vi "Go.vi"(9 "Timing Data":T1(array[cluster]), 10 "Control In":T2={"I-O.lvclass"=refnum, "Gantry"=refnum, "Dispenser"="COM1"}, 11 "C4 Dispense in":refnum<class "Iterative Dispense.lvclass">) -> (2 "Control Out":T2={"I-O.lvclass"=refnum, "Gantry"=refnum, "Dispenser"="COM1"}, 3 "C4 Dispense Out":refnum<class "Iterative Dispense.lvclass">)   [LabVIEW 2020, in "Iterative Dispense.lvclass"]
uses:
  Iterative Dispense.lvclass
  Controller/Controllers.ctl
  Controller/I-O/I-O.lvclass
  C:/Program Files (x86)/Aerotech/A3200/LabVIEW/2010/Bin/Aerotech.A3200.dll
  Program Files (x86)/Aerotech/A3200/LabVIEW/2010/Bin/Aerotech.A3200.dll
  Iterative Dispense.lvclass/Iterative Dispense.ctl
  Controller/Motion/A3200/A3200.lvclass
  Controller/Dispenser/Dispenser.lvclass
  Controller/Motion/Motion.lvclass
  Controller/Controller.lvclass
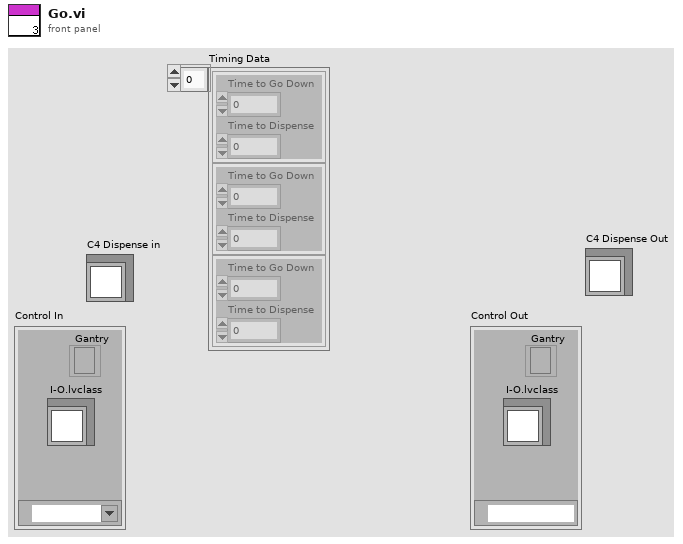
[diagram p1: front panel]
types:
  T1 = cluster{"Time to Go Down":i32, "Time to Dispense":i32}[]
  T2 = typedef "Controller.lvclass/Controllers.ctl" = cluster{"I-O.lvclass":refnum<class "I-O.lvclass">, "Gantry":refnum<k24>, "Dispenser":refnum<visa-resource-name>}
  T3 = typedef "Iterative Dispense.lvclass/Glue Step Enum.ctl" = enum16{"Baseplate to Kapton", "Kapton to Sensor"}
  T4 = cluster{"Time to Go Down":dbl, "Time to Dispense":dbl}
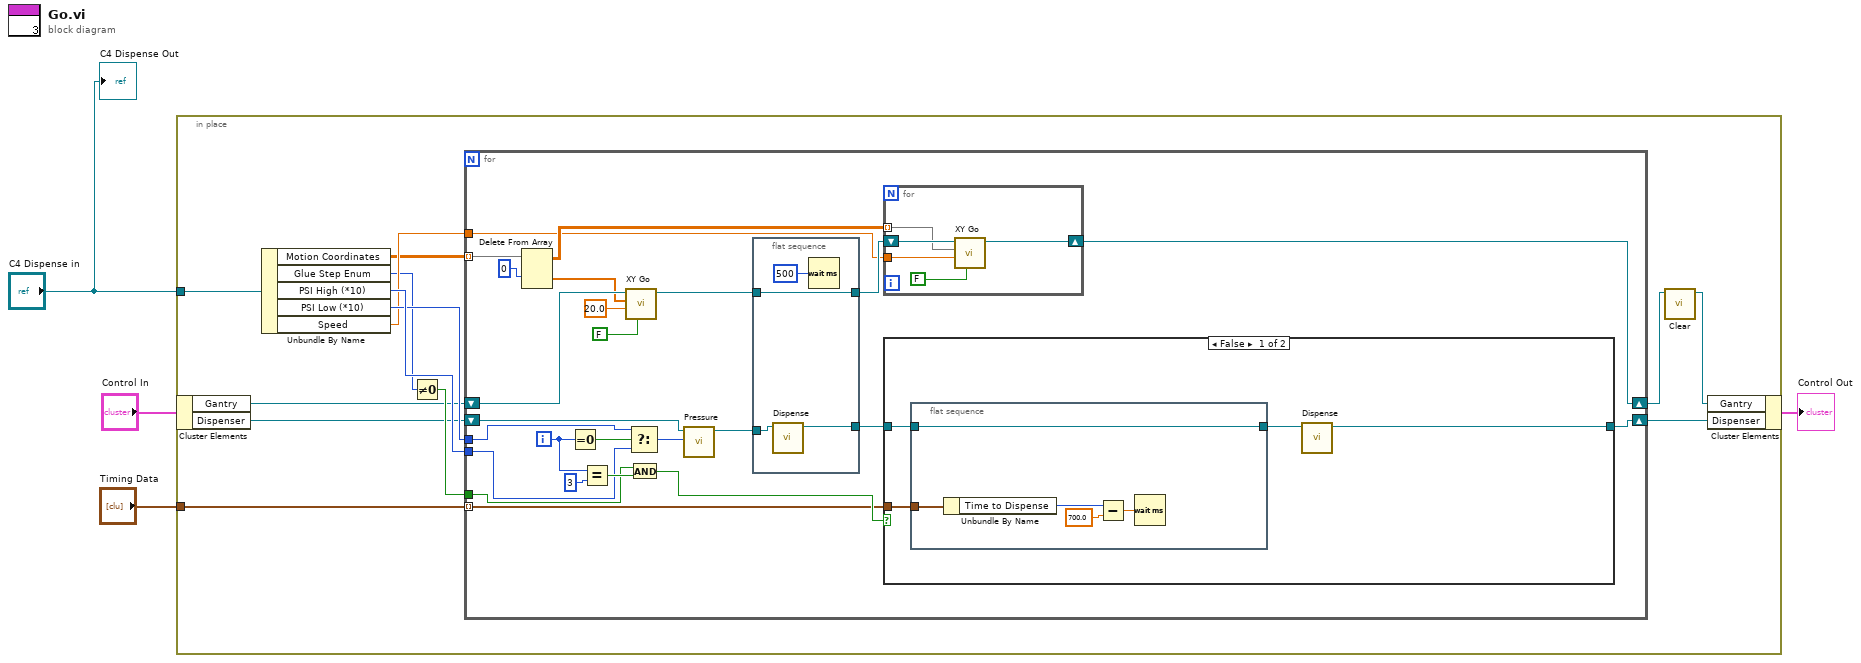
[diagram p0: block diagram]
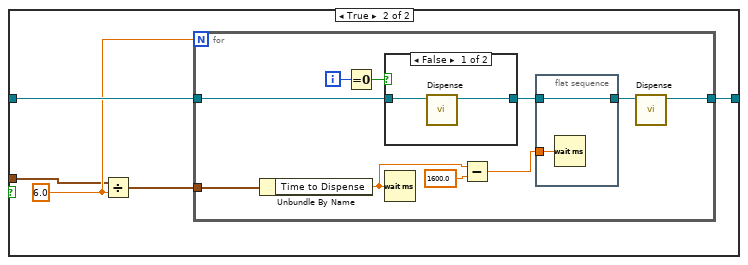
[diagram p2: hidden frame]
diagram:
  n1 = in-place {
    in-place-border: "C4 Dispense in" -> [w16]
    in-place-border: "Timing Data" -> [w12]
    n2 = in-place-cluster #1("Control In") -> ("Gantry"=w9:refnum<k24>, "Dispenser"=w7:refnum<visa-resource-name>)
    n3 = Unbundle By Name(w16) -> ("Motion Coordinates"=w11:dbl[][][], "Glue Step Enum"=w10:T3, "PSI High (*10)"=w15:i32, "PSI Low (*10)"=w14:i32, "Speed"=w13:dbl)
    n4 = Not Equal To 0?(x=w10) -> (x != 0?=w17:bool)
    n5 = for {
      tunnel: w11 -> [w38] mode=indexing
      tunnel: w17 -> [w32]
      tunnel: w13 -> [w30]
      tunnel: w12 -> [w29] mode=indexing
      tunnel: w14 -> [w28]
      tunnel: w15 -> [w27]
      shift-right: [w42] -> w6
      shift-left: w9 -> [w23]
      shift-right: [w39] -> w8
      shift-left: w7 -> [w19]
      i -> [w24]
      # "Executes C4 Symmetric Motion"
      n6 = Delete From Array(array=w38, index (row)=0) -> (deleted portion=w21:dbl[], array with subset deleted=w36:dbl[][])  [unwired: 2 in]
      n7 = Equal To 0?(x=w24) -> (x = 0?=w31:bool)
      n8 = Equal?(x=w24, y=3) -> (x = y?=w40:bool)
      n9 = call "XY Go.vi"("return immediately"=FALSE, "Speed"=20.0 ("speed"), "XY In"=w21, "Gantry In"=w23) -> ("Gantry Out"=w22:refnum<k24>)  [unwired: 5 in, 2 out]
      n10 = Select(t=w28, s=w31, f=w27) -> (s? t:f=w25:i32)
      n11 = And(x=w32, y=w40) -> (x .and. y?=w33:bool)
      n12 = call "Pressure.vi"("Pressure"=w25, "VISA resource name"=w19) -> ("VISA resource name out"=w26:refnum<visa-resource-name>)  [unwired: 8 in, 1 out]
      n13 = flat-sequence {
        tunnel: w26 -> [w72]
        tunnel: w22 -> [w74]
        tunnel: [w74] -> w35
        tunnel: [w73] -> w34
        frame #0 {
          n14 = call "Dispense.vi"("Dispenser In"=w72) -> ("Dispenser Out"=w73:refnum<visa-resource-name>)  [unwired: 9 in, 1 out]
          n15 = Wait (ms)(milliseconds to wait=u32 500) -> ()  [unwired: 1 out]
        }
      }
      n16 = for {
        tunnel: w30 -> [w77]
        tunnel: w36 -> [w78] mode=indexing
        shift-right: [w79] -> w42
        shift-left: w35 -> [w80]
        n17 = call "XY Go.vi"("return immediately"=FALSE, "Speed"=w77, "XY In"=w78, "Gantry In"=w80) -> ("Gantry Out"=w79:refnum<k24>)  [unwired: 5 in, 2 out]
      }
      n18 = case shown="False" w33 {
        tunnel: w29 -> [w46 w52]
        tunnel: w34 -> [w45 w55]
        tunnel: [w44 w54] -> w39
        frame False {
          n19 = flat-sequence {
            tunnel: w45 -> [w49]
            tunnel: w46 -> [w48]
            tunnel: [w49] -> w43
            frame #0 {
              n20 = Unbundle By Name(w48) -> ("Time to Dispense"=w47:i32)
              n21 = Subtract(x=w47, y=700.0) -> (x-y=w51:dbl)
              n22 = Wait (ms)(milliseconds to wait=w51) -> ()  [unwired: 1 out]
            }
          }
          n23 = call "Dispense.vi"("Dispenser In"=w43) -> ("Dispenser Out"=w44:refnum<visa-resource-name>)  [unwired: 9 in, 1 out]
        }
        frame True {
          w53 = 6.0 ("y")
          # "Leaves Space for Silver Epoxy"
          n24 = Divide(x=w52, y=w53) -> (x/y=w56:T4)
          n25 = for {
            N: w53 -> [_]
            tunnel: w56 -> [w58]
            tunnel: w55 -> [w64]
            tunnel: [w60] -> w54
            i -> [w62]
            n26 = Unbundle By Name(w58) -> ("Time to Dispense"=w57:dbl)
            n27 = Equal To 0?(x=w62) -> (x = 0?=w61:bool)
            n28 = case shown="False" w61 {
              tunnel: w64 -> [w67 w69]
              tunnel: [w68 w69] -> w63
              frame False {
                n29 = call "Dispense.vi"("Dispenser In"=w67) -> ("Dispenser Out"=w68:refnum<visa-resource-name>)  [unwired: 9 in, 1 out]
              }
              frame True {
              }
            }
            n30 = Wait (ms)(milliseconds to wait=w57) -> ()  [unwired: 1 out]
            n31 = Subtract(x=w57, y=1600.0) -> (x-y=w65:dbl)
            n32 = flat-sequence {
              tunnel: w65 -> [w71]
              tunnel: w63 -> [w70]
              tunnel: [w70] -> w59
              frame #0 {
                n33 = Wait (ms)(milliseconds to wait=w71) -> ()  [unwired: 1 out]
              }
            }
            n34 = call "Dispense.vi"("Dispenser In"=w59) -> ("Dispenser Out"=w60:refnum<visa-resource-name>)  [unwired: 9 in, 1 out]
          }
        }
      }
    }
    n35 = call "Clear.vi"("Gantry In"=w6) -> ("Gantry Out"=w5:refnum<k24>)  [unwired: 9 in, 1 out]
    n36 = in-place-cluster #1("Gantry"=w5, "Dispenser"=w8) -> (→"Control Out":T2)
  }
  "C4 Dispense Out" <- "C4 Dispense in"
